vi "Pop-up wait prompt with cancel button.vi"(4 "Show Cancel button? (T)":bool=TRUE, 6 "Disable? (F)":bool, 8 "error in":errorcluster, 9 "Prompt Text":string, 11 "Control":enum16{"Open", "Close", "Status", "No Change"}(ring)) -> (0 "error out":errorcluster, 1 "Cancel":bool)   [LabVIEW 2013]
doc: "If there is no error in, this vi will either open or close the calling panel which displays a prompt to wait. The input control determines whether the panel is opened or closed. Typically called before intensive processing with control=open and after with control = close.\n\nClose action ignores error in."
uses:
  <vilib>/Utility/miscctls.llb/LVPointTypeDef.ctl
panel:
  in  "Cancel":bool
  out "Prompt":string
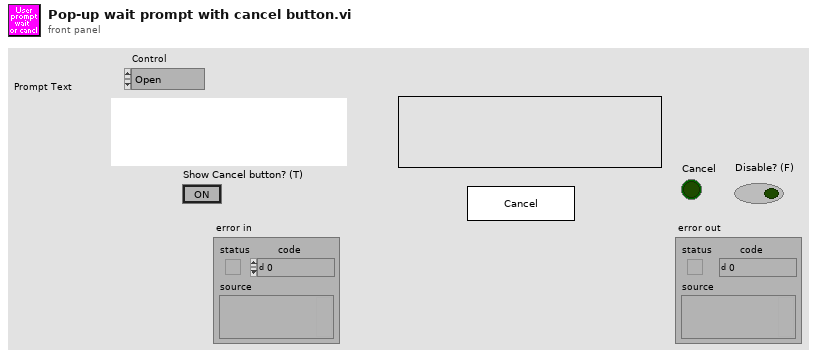
[diagram p1: front panel]
types:
  T1 = typedef "LVPointTypeDef.ctl" = cluster{"Horizontal":i16, "Vertical":i16}
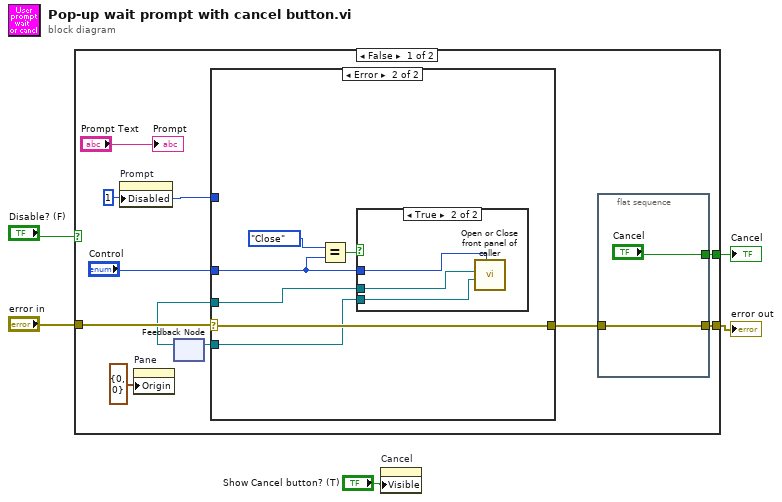
[diagram p0: block diagram]
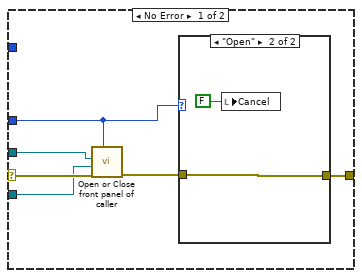
[diagram p2: hidden frame]
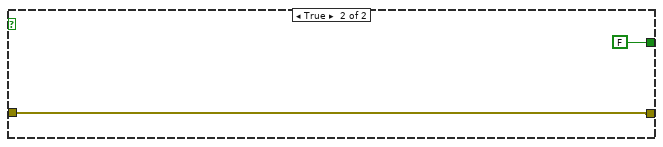
[diagram p5: hidden frame]
diagram:
  n1 = case shown="False" "Disable? (F)" {
    tunnel: [w12 w38] -> w5
    tunnel: "error in" -> [w10 w38]
    tunnel: [w8 FALSE ("Cancel")] -> w2
    frame False {
      w14 = u8 1 ("Write Attribute")
      n2 = property on="Prompt" class="Str"("Disabled"=w14) -> ()  [unwired: 2 in, 2 out]
      n3 = property on="Pane" class="Pane"("Origin"=T1 {"Horizontal"=0, "Vertical"=0}) -> ()  [unwired: 2 in, 2 out]
      n4 = feedback #1() -> (w6:refnum<vi>)  [unwired: 1 in]
      n5 = case shown="Error" w10 {
        selector: w10 -> [w21 w32]
        tunnel: [w22 w32] -> w11
        tunnel: "Control" -> [w20 w30]
        tunnel: w14 -> [_ _]
        tunnel: [w19 w28] -> w7
        tunnel: w6 -> [w18 w27]
        frame No Error {
          n6 = call "Open or Close front panel of caller.vi"("Control"=w20, "error in (no error)"=w21, "VI Refnum in"=w18) -> ("error out"=w23:errorcluster, "VI Refnum out"=w19:refnum<vi>)  [unwired: 2 in, 3 out]
          n7 = case shown="\"Open\"" w20 {
            tunnel: w23 -> [w24 w25]
            tunnel: [w24 w25] -> w22
            frame Default {
            }
            frame "Open" {
              n8 = local write "Cancel"(FALSE ("Cancel")) -> ()
            }
          }
        }
        frame Error {
          n9 = Equal?(x=enum16{"Open", "Close", "Status", "No Change"}."Close", y=w30) -> (x = y?=w29:bool)
          n10 = case shown="True" w29 {
            tunnel: w30 -> [_ w36]
            tunnel: [w33 w35] -> w28
            tunnel: w27 -> [w33 w34]
            frame False {
            }
            frame True {
              n11 = call "Open or Close front panel of caller.vi"("Control"=w36, "VI Refnum in"=w34) -> ("VI Refnum out"=w35:refnum<vi>)  [unwired: 3 in, 4 out]
            }
          }
        }
      }
      n12 = feedback-in #1(w7) -> ()
      n13 = flat-sequence {
        tunnel: [w17] -> w12
        tunnel: w11 -> [w17]
        tunnel: ["Cancel"] -> w8
        frame #0 {
        }
      }
      "Prompt" <- "Prompt Text"
    }
    frame True {
    }
  }
  "error out" <- w5
  "Cancel" <- w2
  n14 = property on="Cancel" class="Bool (strict)"("Visible"="Show Cancel button? (T)") -> ()  [unwired: 2 in, 2 out]
